vi "active_index_to_crate_card_chan.vi"(8 "Channels in Active":T1[](array[typedef]) {"Card.Channel" format="%.2f"}, 11 "Index":i32) -> (1 "Card":i32, 2 "Channel":i32, 3 "Crate":i32)   [LabVIEW 2018]
uses:
  subvis/channel.ctl
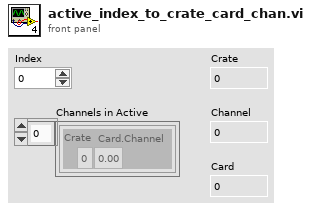
[diagram p1: front panel]
types:
  T1 = typedef "channel.ctl" = cluster{" Card.Channel":dbl, "Crate":i32}
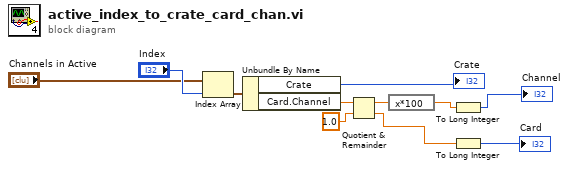
[diagram p0: block diagram]
diagram:
  n1 = Index Array(array="Channels in Active", index="Index") -> (element=w9:T1)
  n2 = Unbundle By Name(w9) -> ("Crate"=→"Crate":i32, "Card.Channel"=w10:dbl)
  n3 = Quotient & Remainder(x=w10, y=1.0) -> (x-y*floor(x/y)=w8:dbl, floor(x/y)=w4:dbl)
  n4 = expression code="x*100"(w8) -> (w2:dbl)
  n5 = To Long Integer(number=w2) -> (32bit integer=→"Channel":i32)
  n6 = To Long Integer(number=w4) -> (32bit integer=→"Card":i32)
